vi "Joystick Drive.vi"   [LabVIEW 2014]
types:
  T1 = cluster{"Buttons":cluster{"1":bool, "2":bool, "3":bool, "4":bool, "5":bool, "6":bool, "7":bool, "8":bool, "9":bool, "10":bool}, "Axes":cluster{"X":dbl, "Y":dbl, "Throttle":dbl}}
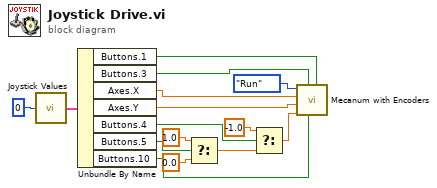
[diagram p0: block diagram]
diagram:
  n1 = call "Joystick Values.vi"("Joystick Index"=0) -> ("Joystick"=w13:T1)
  n2 = Unbundle By Name(w13) -> ("Buttons.1"=w1:bool, "Buttons.3"=w2:bool, "Axes.X"=w12:dbl, "Axes.Y"=w11:dbl, "Buttons.4"=w9:bool, "Buttons.5"=w8:bool, "Buttons.10"=w3:bool)
  n3 = Select(t=1.0, s=w8, f=0.0) -> (s? t:f=w6:dbl)
  n4 = Select(t=-1.0, s=w9, f=w6) -> (s? t:f=w5:dbl)
  n5 = call "Mecanum with Encoders.vi"("Slow?"=w1, "Reset"=w3, "Fast?"=w2, "Turn"=w5, "Forward/Backward"=w11, "Strafe"=w12, "Mode"=enum8{"Start", "Run", "Finish"}."Run") -> ()  [unwired: 3 in, 1 out]
